vi "Read Project Data ref.vi"(8 "error in (no error)":errorcluster, 11 "UI Wizard in":refnum<class "UI Wizard.lvclass">) -> (0 "error out":errorcluster, 2 "Project Data ref":refnum<data-value>, 3 "UI Wizard out":refnum<class "UI Wizard.lvclass">)   [LabVIEW 2013, in "SET Project Editor.lvlib" / "UI Wizard.lvclass"]
uses:
  UI Wizard.lvclass
  SET Project Data/Project Data Class/Project Data.lvclass
  UI Wizard.lvclass/UI Wizard.ctl
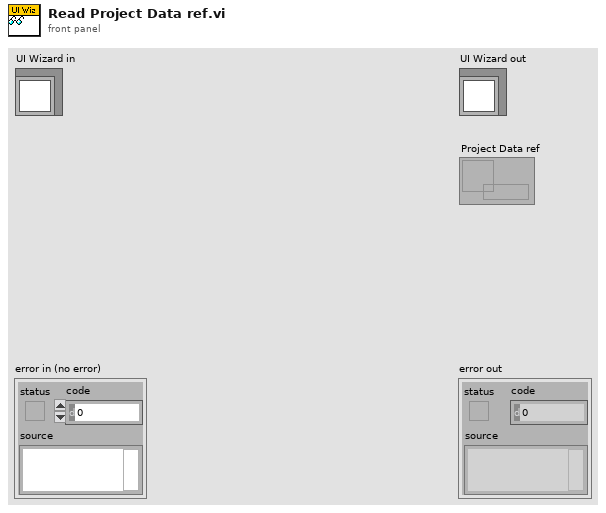
[diagram p1: front panel]
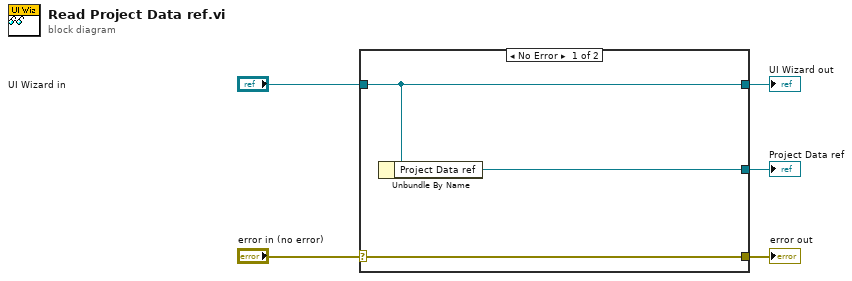
[diagram p0: block diagram]
diagram:
  n1 = case shown="No Error" "error in (no error)" {
    selector: "error in (no error)" -> [w8 w9]
    tunnel: [w8 w9] -> w4
    tunnel: [w7 w10] -> w2
    tunnel: "UI Wizard in" -> [w7 w10]
    tunnel: [w6 _] -> w1
    frame No Error {
      n2 = Unbundle By Name(w7) -> ("Project Data ref"=w6:refnum<data-value>)
    }
    frame Error {
    }
  }
  "error out" <- w4
  "UI Wizard out" <- w2
  "Project Data ref" <- w1
